vi "View Prior Tab.vi"(7 "QRD":T1, 8 "error in":errorcluster) -> (0 "error out":errorcluster, 5 "QRD Out":T1)   [LabVIEW 2025]
uses:
  Controls/Queues-Refs-Data.ctl
  Builds/Queue Wrappers.lvlibp/Q Packet.ctl
  Builds/Queue Wrappers.lvlibp
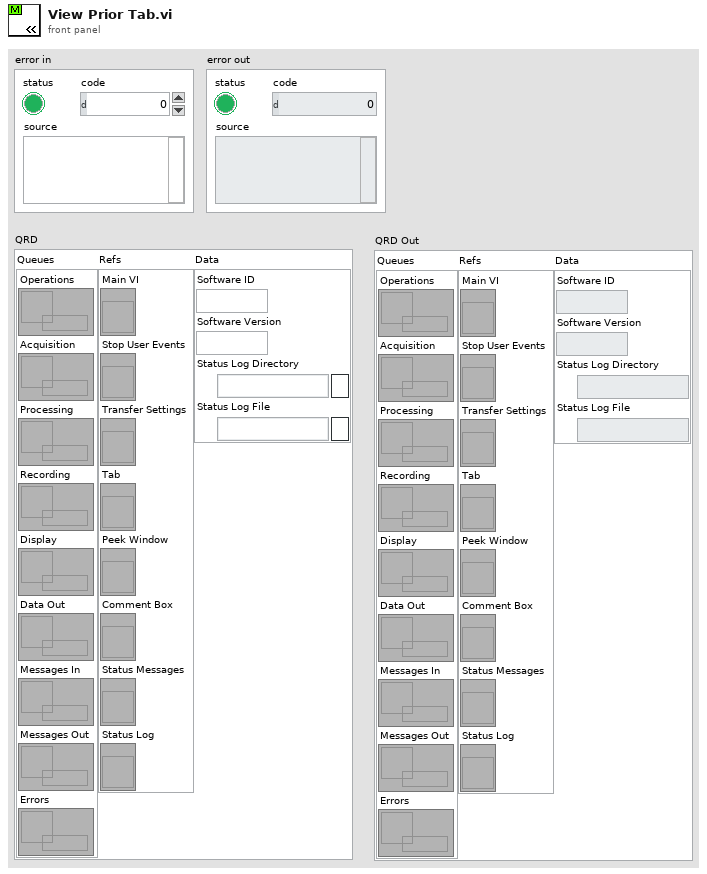
[diagram p1: front panel]
types:
  T1 = typedef "Queues-Refs-Data.ctl" = cluster{"Queues":cluster{"Operations":refnum<queue>, "Acquisition":refnum<queue>, "Processing":refnum<queue>, "Recording":refnum<queue>, "Display":refnum<queue>, "Data Out":refnum<queue>, "Messages In":refnum<queue>, "Messages Out":refnum<queue>, "Errors":refnum<queue>}, "Refs":cluster{"Main VI":refnum<vi>, "Stop User Events":refnum<vi>, "Transfer Settings":refnum<vi>, "Tab":refnum<vi>, "Peek Window":refnum<vi>, "Comment Box":refnum<vi>, "Status Messages":refnum<vi>, "Status Log":refnum<vi>}, "Data":cluster{"Software ID":string, "Software Version":string, "Status Log Directory":path, "Status Log File":path}}
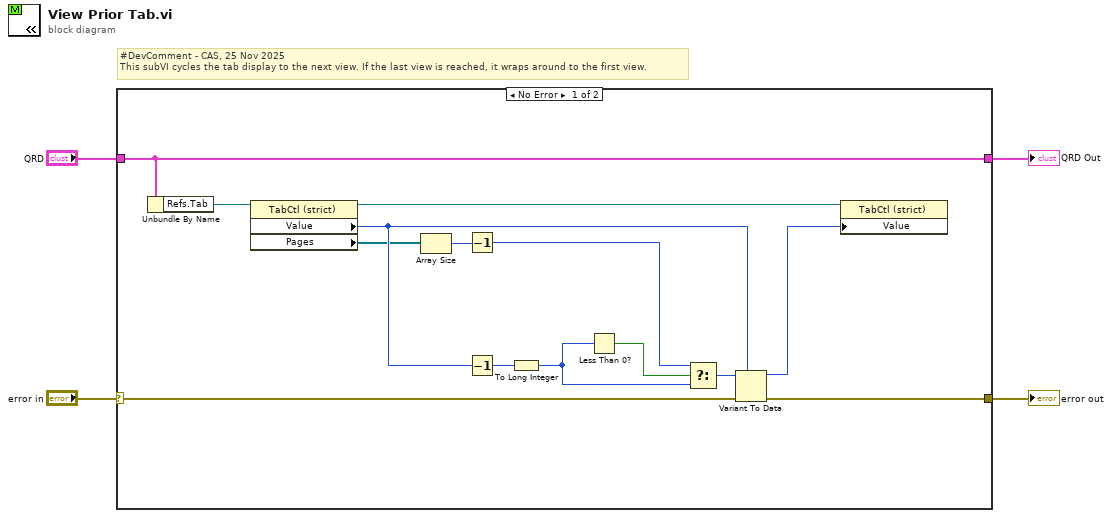
[diagram p0: block diagram]
diagram:
  # "#DevComment - CAS, 25 Nov 2025\nThis subVI cycles the tab display to the next view. If the last view is reached, it wraps around to the first view."
  n1 = case shown="No Error" "error in" {
    selector: "error in" -> [w11 w19]
    tunnel: [w10 w19] -> w3
    tunnel: "QRD" -> [w9 w20]
    tunnel: [w9 w20] -> w1
    frame No Error {
      n2 = Unbundle By Name(w9) -> ("Refs.Tab"=w18:refnum<vi>)
      n3 = property class="TabCtl (strict)"(reference=w18) -> (reference out=w17:refnum<vi>, "Value"=w13:enum32{"Page 1", "Page 2", "Status Log"}, "Pages"=w8:refnum<vi>[])  [unwired: 1 in, 1 out]
      n4 = Array Size(array=w8) -> (size(s)=w7:i32)
      n5 = Decrement(x=w7) -> (x-1=w6:i32)
      n6 = Decrement(x=w13) -> (x-1=w16:enum32{"Page 1", "Page 2", "Status Log"})
      n7 = To Long Integer(number=w16) -> (32bit integer=w5:i32)
      n8 = Less Than 0?(x=w5) -> (x < 0?=w15:bool)
      n9 = Select(t=w6, s=w15, f=w5) -> (s? t:f=w14:i32)
      n10 = Variant To Data(error in=w11, type=w13, Variant=w14) -> (data=w12:enum32{"Page 1", "Page 2", "Status Log"}, error out=w10:errorcluster)
      n11 = property class="TabCtl (strict)"(reference=w17, "Value"=w12) -> ()  [unwired: 1 in, 2 out]
    }
    frame Error {
    }
  }
  "error out" <- w3
  "QRD Out" <- w1
